vi "Weight.vi"(10 "待处理":string, 11 "read buffer":string) -> (2 "result string":string, 3 "数值":dbl format="%#.3f")   [LabVIEW 2014]
panel:
  out "连接的字符串":string
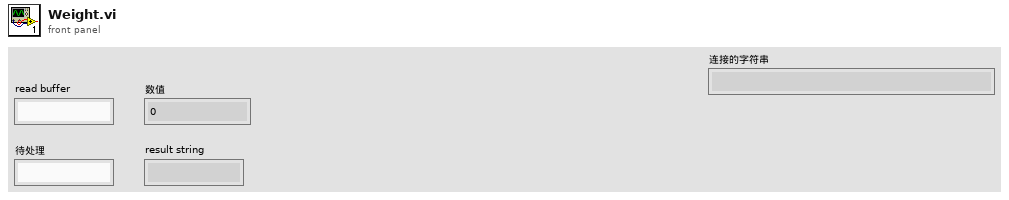
[diagram p1: front panel]
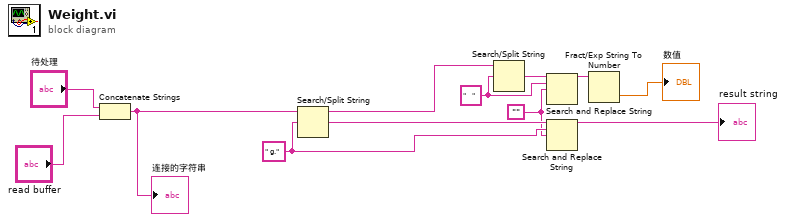
[diagram p0: block diagram]
diagram:
  w2 = "   " ("搜索字符串/字符(-)")
  w3 = ""
  w7 = " g." ("搜索字符串/字符(-)")
  n1 = Concatenate Strings("待处理", "read buffer") -> (w11:string)
  "连接的字符串" <- w11
  n2 = Search/Split String(string=w11, search string/char (-)=w7) -> (substring before match=w8:string, match + rest of string=w6:string)  [unwired: 1 in, 1 out]
  n3 = Search/Split String(string=w8, search string/char (-)=w2) -> (match + rest of string=w1:string)  [unwired: 1 in, 2 out]
  n4 = Search and Replace String(input string=w1, search string=w2, replace string=w3) -> (result string=w4:string)  [unwired: 5 in, 3 out]
  n5 = Search and Replace String(input string=w6, search string=w7, replace string=w3) -> (result string=→"result string":string)  [unwired: 5 in, 3 out]
  n6 = Fract/Exp String To Number(string=w4) -> (number=→"数值":dbl)  [unwired: 3 in, 1 out]
